vi "Program for lab 2.vi"() -> ()   [LabVIEW 2010]
uses:
  <vilib>/Utility/file.llb/Write To Spreadsheet File (DBL).vi
  <vilib>/Analysis/NI_AALBase.lvlib
panel:
  in  "Switch to\nsave output":bool
  out "Waveform Graph":dbl[](graph)
  out "Histogram":T1(graph)
  out "Random\nnumbers":dbl[](array[numeric])
  in  "Number of\nrandom numbers":i32
  in  "Target random number":dbl
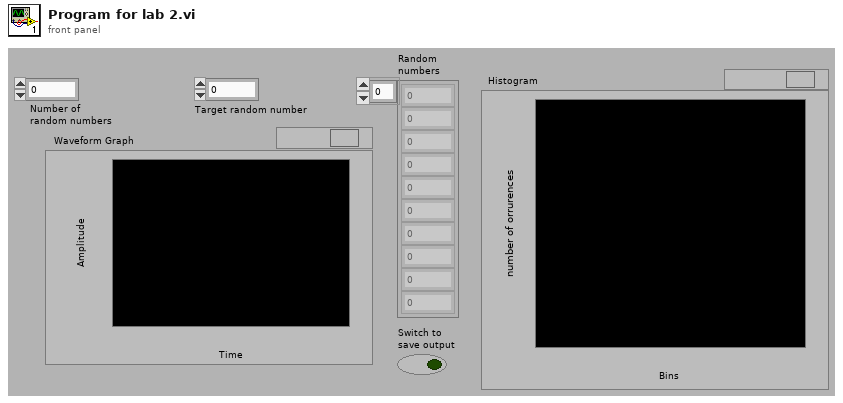
[diagram p1: front panel]
types:
  T1 = cluster{"X Values":dbl[], "Histogram: h(x)":i32[]}
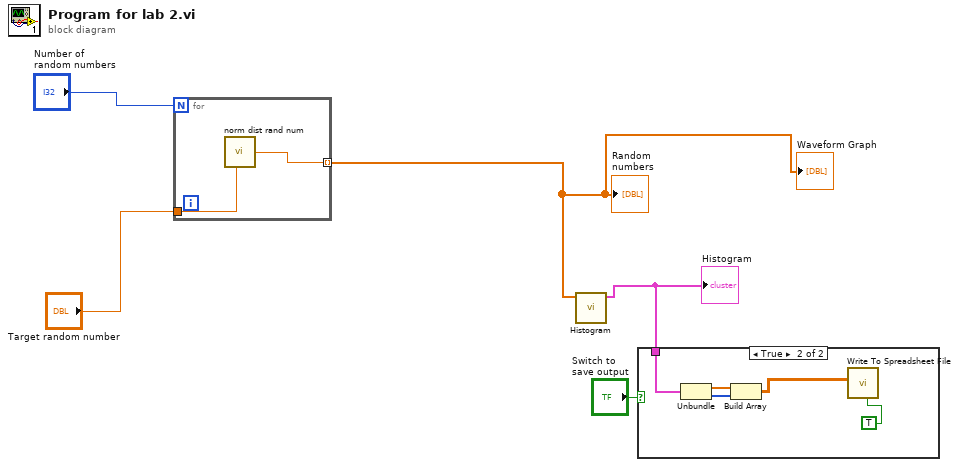
[diagram p0: block diagram]
diagram:
  n1 = for {
    N: "Number of\nrandom numbers" -> [_]
    tunnel: "Target random number" -> [w7]
    tunnel: [w6] -> w3 mode=indexing
    n2 = call "norm dist rand num.vi"("Numeric 2"=w7) -> ("Numeric"=w6:dbl)
  }
  "Random\nnumbers" <- w3
  "Waveform Graph" <- w3
  n3 = call <vilib>:"Histogram.vi"("X"=w3) -> ("Histogram Graph"=w1:T1)  [unwired: 7 in, 3 out]
  "Histogram" <- w1
  n4 = case shown="True" "Switch to\nsave output" {
    tunnel: w1 -> [_ w12]
    frame False {
    }
    frame True {
      n5 = Unbundle(w12) -> ("X Values"=w11:dbl[], "Histogram: h(x)"=w10:i32[])
      n6 = Build Array(w11, w10) -> (w9:dbl[][])
      n7 = call-poly <vilib>:"Write To Spreadsheet File.vi"("transpose? (no:F)"=TRUE, "2D data"=w9) -> ()  [unwired: 6 in, 1 out]
    }
  }
